vi "termometer delay.vi"() -> ()   [LabVIEW 2023]
panel:
  in  "Thermometer":dbl(slide) scale=0.0..100.0
  out "Numeric":i32
  out "Boolean":bool
  in  "stop":bool
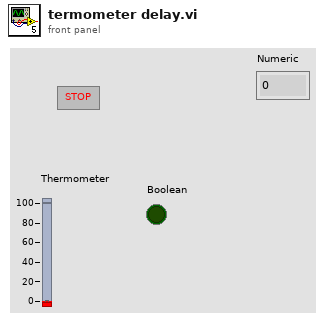
[diagram p1: front panel]
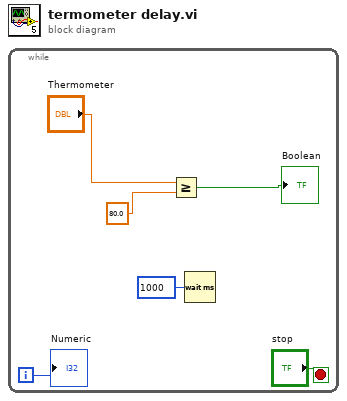
[diagram p0: block diagram]
diagram:
  n1 = while {
    i -> [w4]
    stop <- "stop" stop-if-true
    n2 = Greater Or Equal?(x="Thermometer", y=80.0 ("x")) -> (x >= y?=→"Boolean":bool)
    n3 = Wait (ms)(milliseconds to wait=u32 1000) -> ()  [unwired: 1 out]
    "Numeric" <- w4
  }
